vi "PruneAutosaves.vi"(8 "error in":errorcluster, 10 "Autosave Depth":i32=20, 11 "Autosave Directory":path) -> (0 "error out":errorcluster, 1 "Current Autosaves":path[](array[path]), 2 "Deleted Autosaves":path[](array[path]), 4 "Deletion Errors":errorcluster[](array[cluster]), 6 "Error Deleting Autosaves":path[](array[path]))   [LabVIEW 2013]
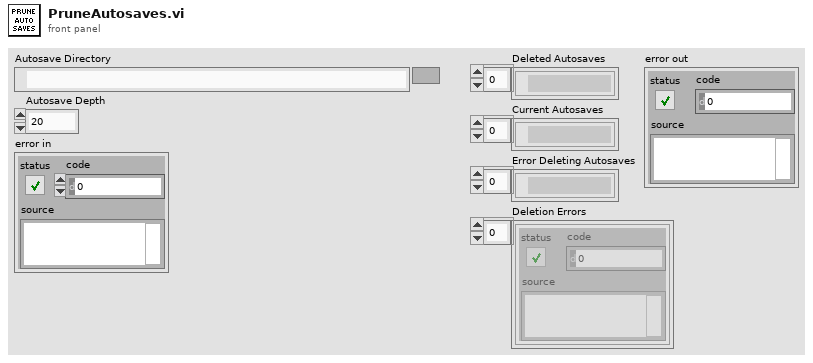
[diagram p1: front panel]
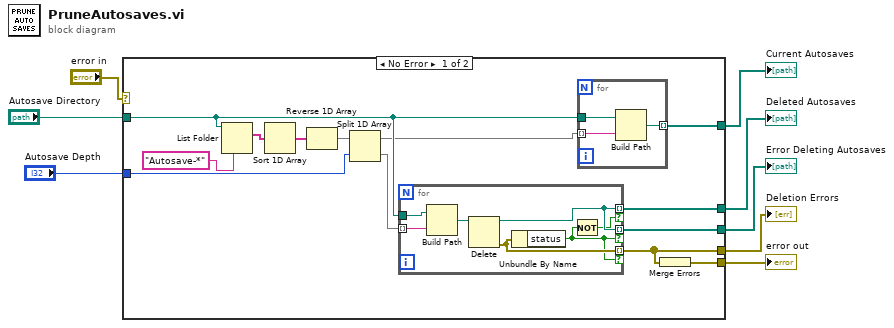
[diagram p0: block diagram]
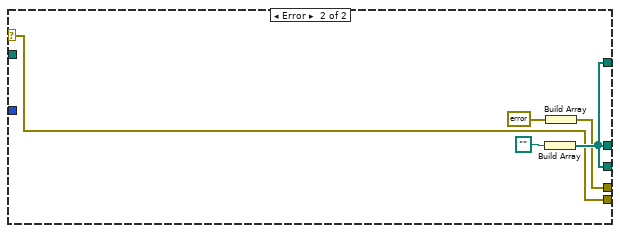
[diagram p2: hidden frame]
diagram:
  n1 = case shown="No Error" "error in" {
    selector: "error in" -> [_ w34]
    tunnel: "Autosave Depth" -> [w9 _]
    tunnel: [w18 w35] -> w7
    tunnel: "Autosave Directory" -> [w17 _]
    tunnel: [w16 w35] -> w5
    tunnel: [w15 w35] -> w4
    tunnel: [w14 w34] -> w1
    tunnel: [w13 w32] -> w2
    frame No Error {
      n2 = List Folder(path=w17, pattern="Autosave-*") -> (filenames=w20:string[])  [unwired: 2 in, 3 out]
      n3 = Sort 1D Array(array=w20) -> (sorted array=w19:string[])
      n4 = Reverse 1D Array(array=w19) -> (reversed array=w12:string[])
      n5 = Split 1D Array(array=w12, index=w9) -> (first subarray=w11:string[], second subarray=w10:string[])
      n6 = for {
        tunnel: w10 -> [w30] mode=indexing
        tunnel: w17 -> [w31]
        tunnel: [w28] -> w18 mode=indexing if=w26
        tunnel: [w28] -> w15 mode=indexing if=w25
        tunnel: [w27] -> w13 mode=indexing if=w25
        n7 = Build Path(base path=w31, name or relative path=w30) -> (appended path=w29:path)
        n8 = Delete(path (use dialog)=w29) -> (deleted path=w28:path, error out=w27:errorcluster)  [unwired: 4 in, 1 out]
        n9 = Unbundle By Name(w27) -> ("status"=w25:bool)
        n10 = Not(x=w25) -> (.not. x?=w26:bool)
      }
      n11 = for {
        tunnel: w11 -> [w23] mode=indexing
        tunnel: w17 -> [w24]
        tunnel: [w22] -> w16 mode=indexing
        n12 = Build Path(base path=w24, name or relative path=w23) -> (appended path=w22:path)
      }
      n13 = Merge Errors(w13) -> (w14:errorcluster)
    }
    frame Error {
      n14 = Build Array(path "") -> (w35:path[])
      n15 = Build Array(errorcluster {"status"=FALSE, "code"=0, "source"=""} ("error constant")) -> (w32:errorcluster[])
    }
  }
  "Deleted Autosaves" <- w7
  "Current Autosaves" <- w5
  "Error Deleting Autosaves" <- w4
  "Deletion Errors" <- w2
  "error out" <- w1
